vi "LOC subReadWriteVIStringINIKeys(RadioButtons).vi"(4 "Mode":enum16{"Read", "Write"}(ring), 5 "Section":string, 6 "error in (no error)":errorcluster, 8 "ConfigFileRefnum":T1, 9 "ControlRefnum":refnum<vi>) -> (0 "error out":errorcluster)   [LabVIEW 2020, in "Localization_Tools.lvlib"]
uses:
  Localization_Tools.lvlib
  <vilib>/Utility/config.llb/Config Data RefNum.ctl
  <vilib>/Utility/config.llb/NI_LVConfig.lvlib
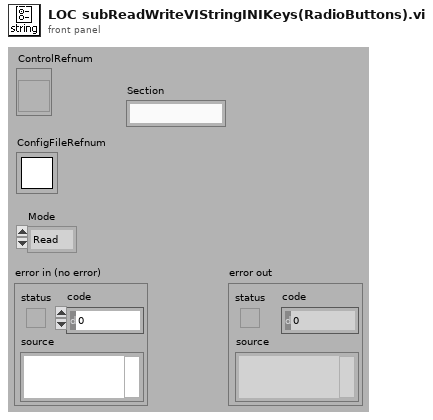
[diagram p1: front panel]
types:
  T1 = typedef "NI_LVConfig.lvlib/Config Data RefNum.ctl" = refnum<k1>
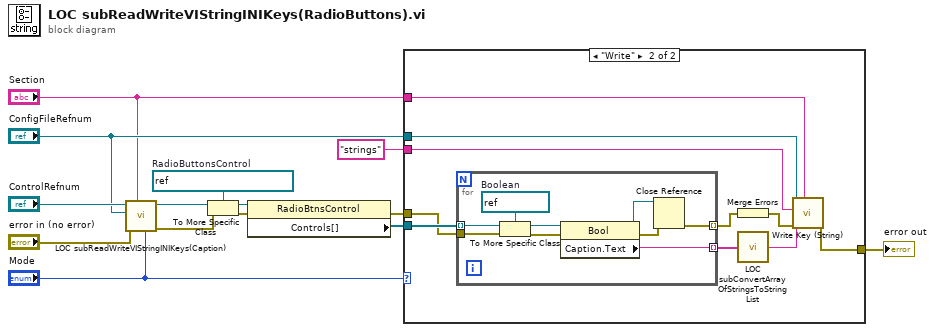
[diagram p0: block diagram]
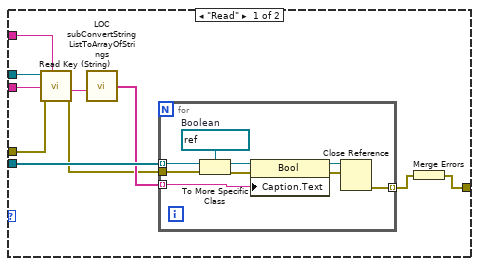
[diagram p2: hidden frame]
diagram:
  w6 = refnum<vi> refnum  # RadioButtonsControl
  n1 = call "LOC subReadWriteVIStringINIKeys(Caption).vi"("Mode"="Mode", "Section"="Section", "error in (no error)"="error in (no error)", "ConfigFileRefnum"="ConfigFileRefnum", "ControlRefnum"="ControlRefnum") -> ("error out"=w7:errorcluster, "dup ControlRefnum"=w8:refnum<vi>)  [unwired: 3 in]
  n2 = To More Specific Class(target class=w6, reference=w8, error in=w7) -> (specific class reference=w5:refnum<vi>, error out=w4:errorcluster)
  n3 = property class="RadioBtnsControl"(reference=w5, error in=w4) -> (error out=w3:errorcluster, "Controls[]"=w2:refnum<vi>[])  [unwired: 1 out]
  n4 = case shown="\"Write\"" "Mode" {
    tunnel: w3 -> [w19 w36]
    tunnel: "ConfigFileRefnum" -> [w24 w43]
    tunnel: "Section" -> [w23 w41]
    tunnel: "strings" ("key") -> [w22 w42]
    tunnel: [w21 w40] -> w1
    tunnel: w2 -> [w18 w37]
    frame "Read" {
      n5 = call <vilib>:"Read Key (String).vi"("section"=w23, "error in (no error)"=w19, "key"=w22, "refnum"=w24) -> ("error out"=w15:errorcluster, "value"=w20:string)  [unwired: 4 in, 2 out]
      n6 = call "LOC subConvertStringListToArrayOfStrings.vi"("InputString"=w20) -> ("OutputArray"=w17:string[])
      n7 = for {
        tunnel: w18 -> [w31] mode=indexing
        tunnel: w17 -> [w30] mode=indexing
        tunnel: [w25] -> w16 mode=indexing
        tunnel: w15 -> [w29]
        w32 = refnum<vi> refnum  # Boolean
        n8 = To More Specific Class(target class=w32, reference=w31, error in=w29) -> (specific class reference=w33:refnum<vi>, error out=w28:errorcluster)
        n9 = property class="Bool"(reference=w33, error in=w28, "Caption.Text"=w30) -> (reference out=w27:refnum<vi>, error out=w26:errorcluster)
        n10 = Close Reference(reference=w27, error in (no error)=w26) -> (error out=w25:errorcluster)
      }
      n11 = Merge Errors(w16) -> (w21:errorcluster)
    }
    frame "Write" {
      n12 = for {
        tunnel: w37 -> [w50] mode=indexing
        tunnel: [w49] -> w38 mode=indexing
        tunnel: w36 -> [w48]
        tunnel: [w45] -> w35 mode=indexing
        w51 = refnum<vi> refnum  # Boolean
        n13 = To More Specific Class(target class=w51, reference=w50, error in=w48) -> (specific class reference=w52:refnum<vi>, error out=w47:errorcluster)
        n14 = property class="Bool"(reference=w52, error in=w47) -> (reference out=w44:refnum<vi>, error out=w46:errorcluster, "Caption.Text"=w49:string)
        n15 = Close Reference(reference=w44, error in (no error)=w46) -> (error out=w45:errorcluster)
      }
      n16 = Merge Errors(w35) -> (w34:errorcluster)
      n17 = call "LOC subConvertArrayOfStringsToStringList.vi"("InputArray"=w38) -> ("OutputString"=w39:string)
      n18 = call <vilib>:"Write Key (String).vi"("section"=w41, "error in (no error)"=w34, "value"=w39, "key"=w42, "refnum"=w43) -> ("error out"=w40:errorcluster)  [unwired: 4 in, 2 out]
    }
  }
  "error out" <- w1
